vi "CRYPlot Cursor.vi"(9 "Cursor Ref":refnum<vi>, 10 "Graph Ref":refnum<vi>, 11 "Graph Type":string) -> ()   [LabVIEW 2013]
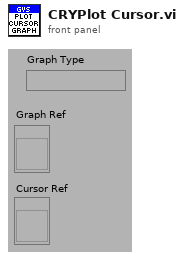
[diagram p1: front panel]
types:
  T1 = typedef "LVPointDoubleTypeDef.ctl" = cluster{"Cursor X":dbl, "Cursor Y":dbl}
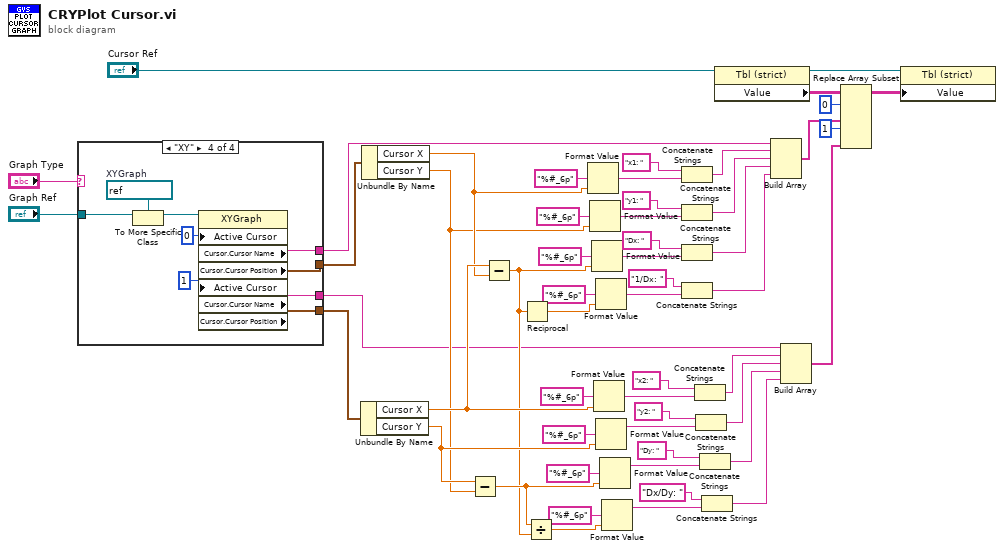
[diagram p0: block diagram]
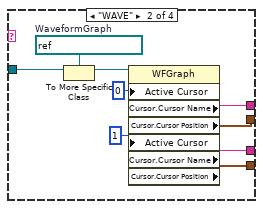
[diagram p3: hidden frame]
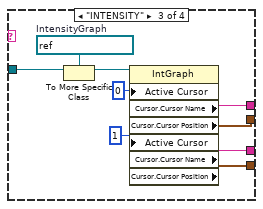
[diagram p4: hidden frame]
diagram:
  n1 = case shown="\"XY\"" "Graph Type" {
    tunnel: "Graph Ref" -> [_ w63 w72 w81]
    tunnel: [_ w58 w67 w76] -> w4
    tunnel: [_ w57 w66 w75] -> w3
    tunnel: [_ w56 w65 w74] -> w2
    tunnel: [_ w55 w64 w73] -> w1
    frame Default {
    }
    frame "WAVE" {
      w62 = refnum<vi> refnum  # WaveformGraph
      n2 = To More Specific Class(target class=w62, reference=w63) -> (specific class reference=w59:refnum<vi>)  [unwired: 1 in, 1 out]
      n3 = property on="Property Node" class="WFGraph"(reference=w59, "Active Cursor"=u32 0, "Active Cursor"=u32 1) -> ("Cursor.Cursor Name"=w58:string, "Cursor.Cursor Position"=w57:T1, "Cursor.Cursor Name"=w56:string, "Cursor.Cursor Position"=w55:T1)  [unwired: 1 in, 2 out]
    }
    frame "INTENSITY" {
      w71 = refnum<vi> refnum  # IntensityGraph
      n4 = To More Specific Class(target class=w71, reference=w72) -> (specific class reference=w68:refnum<vi>)  [unwired: 1 in, 1 out]
      n5 = property on="Property Node" class="IntGraph"(reference=w68, "Active Cursor"=u32 0, "Active Cursor"=u32 1) -> ("Cursor.Cursor Name"=w67:string, "Cursor.Cursor Position"=w66:T1, "Cursor.Cursor Name"=w65:string, "Cursor.Cursor Position"=w64:T1)  [unwired: 1 in, 2 out]
    }
    frame "XY" {
      w80 = refnum<vi> refnum  # XYGraph
      n6 = To More Specific Class(target class=w80, reference=w81) -> (specific class reference=w77:refnum<vi>)  [unwired: 1 in, 1 out]
      n7 = property on="Property Node" class="XYGraph"(reference=w77, "Active Cursor"=u32 0, "Active Cursor"=u32 1) -> ("Cursor.Cursor Name"=w76:string, "Cursor.Cursor Position"=w75:T1, "Cursor.Cursor Name"=w74:string, "Cursor.Cursor Position"=w73:T1)  [unwired: 1 in, 2 out]
    }
  }
  n8 = Unbundle By Name(w1) -> ("Cursor X"=w30:dbl, "Cursor Y"=w28:dbl)
  n9 = Unbundle By Name(w3) -> ("Cursor X"=w29:dbl, "Cursor Y"=w27:dbl)
  n10 = Subtract(x=w28, y=w27) -> (x-y=w13:dbl)
  n11 = Subtract(x=w30, y=w29) -> (x-y=w12:dbl)
  n12 = Reciprocal(x=w12) -> (1/x=w16:dbl)
  n13 = Divide(x=w13, y=w12) -> (x/y=w7:dbl)
  n14 = Format Value(format string="%#_6p", value (0)=w29) -> (output string=w37:string)  [unwired: 1 in]
  n15 = Format Value(format string="%#_6p", value (0)=w27) -> (output string=w38:string)  [unwired: 1 in]
  n16 = Format Value(format string="%#_6p", value (0)=w12) -> (output string=w22:string)  [unwired: 1 in]
  n17 = Format Value(format string="%#_6p", value (0)=w30) -> (output string=w46:string)  [unwired: 1 in]
  n18 = Format Value(format string="%#_6p", value (0)=w16) -> (output string=w17:string)  [unwired: 1 in]
  n19 = Format Value(format string="%#_6p", value (0)=w28) -> (output string=w43:string)  [unwired: 1 in]
  n20 = Format Value(format string="%#_6p", value (0)=w13) -> (output string=w26:string)  [unwired: 1 in]
  n21 = Format Value(format string="%#_6p", value (0)=w7) -> (output string=w10:string)  [unwired: 1 in]
  n22 = Concatenate Strings("x1: " ("string"), w37) -> (w35:string)
  n23 = Concatenate Strings("y1: " ("string"), w38) -> (w36:string)
  n24 = Concatenate Strings("Dx: " ("string"), w22) -> (w19:string)
  n25 = Concatenate Strings("1/Dx: " ("string"), w17) -> (w15:string)
  n26 = Concatenate Strings("x2: " ("string"), w46) -> (w41:string)
  n27 = Concatenate Strings("y2: " ("string"), w43) -> (w42:string)
  n28 = Concatenate Strings("Dy: " ("string"), w26) -> (w23:string)
  n29 = Concatenate Strings("Dx/Dy: " ("string"), w10) -> (w8:string)
  n30 = property on="Property Node" class="Tbl (strict)"(reference="Cursor Ref") -> (reference out=w47:refnum<vi>, "Value"=w49:string[][])  [unwired: 1 in, 1 out]
  n31 = Build Array(w4, w35, w36, w19, w15) -> (w33:string[])
  n32 = Build Array(w2, w41, w42, w23, w8) -> (w34:string[])
  n33 = Replace Array Subset(array=w49, new element #1=w33, index (row) #1=0 ("index (row)"), new element #2=w34, index (row) #2=1 ("index (row)")) -> (w54:string[][])  [unwired: 2 in]
  n34 = property on="Property Node" class="Tbl (strict)"(reference=w47, "Value"=w54) -> ()  [unwired: 1 in, 2 out]
